vi "AoC23-Read input file to 2D array.vi"(11 "input file":path) -> (2 "input text":string, 3 "input":i32[][](array[numeric]))   [LabVIEW 2021]
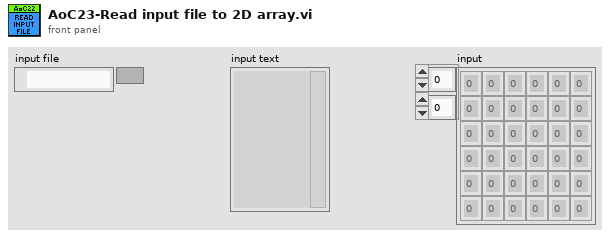
[diagram p1: front panel]
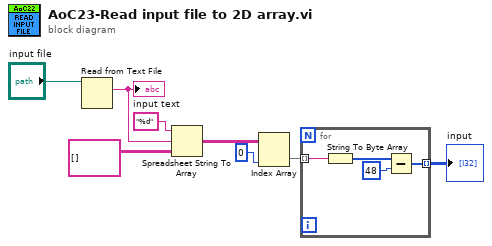
[diagram p0: block diagram]
diagram:
  n1 = Read from Text File(file (use dialog)="input file") -> (text=w8:string)  [unwired: 3 in, 3 out]
  "input text" <- w8
  n2 = Spreadsheet String To Array(format string="%d", spreadsheet string=w8, array type (2D Dbl)=string[][] []) -> (array=w3:string[][])  [unwired: 1 in]
  n3 = Index Array(array=w3, index (col)=0 ("disabled index (col)")) -> (element=w2:string[])  [unwired: 1 in]
  n4 = for {
    tunnel: w2 -> [w9] mode=indexing
    tunnel: [w10] -> w1 mode=indexing
    n5 = String To Byte Array(string=w9) -> (unsigned byte array=w12:u8[])
    n6 = Subtract(x=w12, y=48) -> (x-y=w10:i32[])
  }
  "input" <- w1
